vi "Number list to array.vi"(10 "Full names prefix":string, 11 "Number list":string) -> (1 "Comma-separated list":string, 2 "Full names":string[](array[string]), 3 "Number list array":i32[](array[numeric]), 4 "Channlel set":set{i32}(c389))   [LabVIEW 2024, in "File.lvclass"]
uses:
  File/File Class/File.lvclass
  File/File Class/File.lvclass/File.ctl
panel:
  out "repeat channle numbers":bool
  out "substring":string
  out "number":i32
  out "offset past number":i32
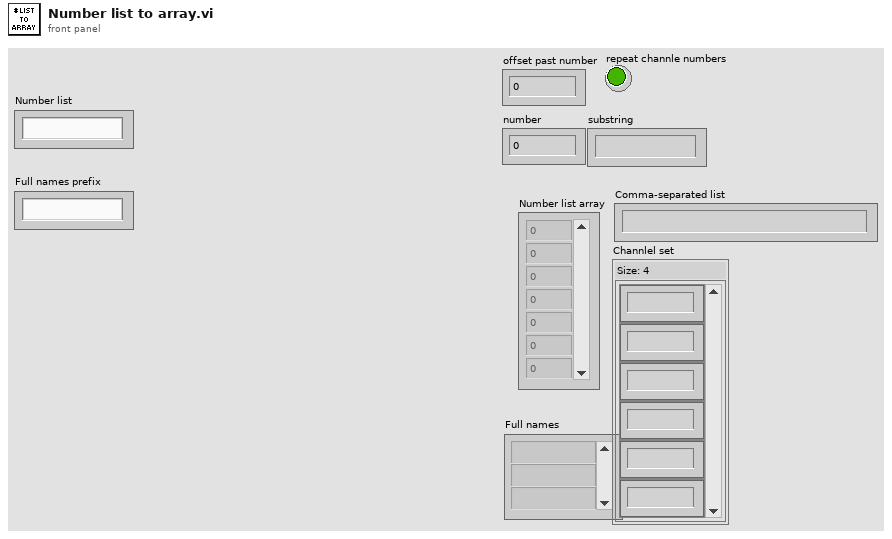
[diagram p1: front panel]
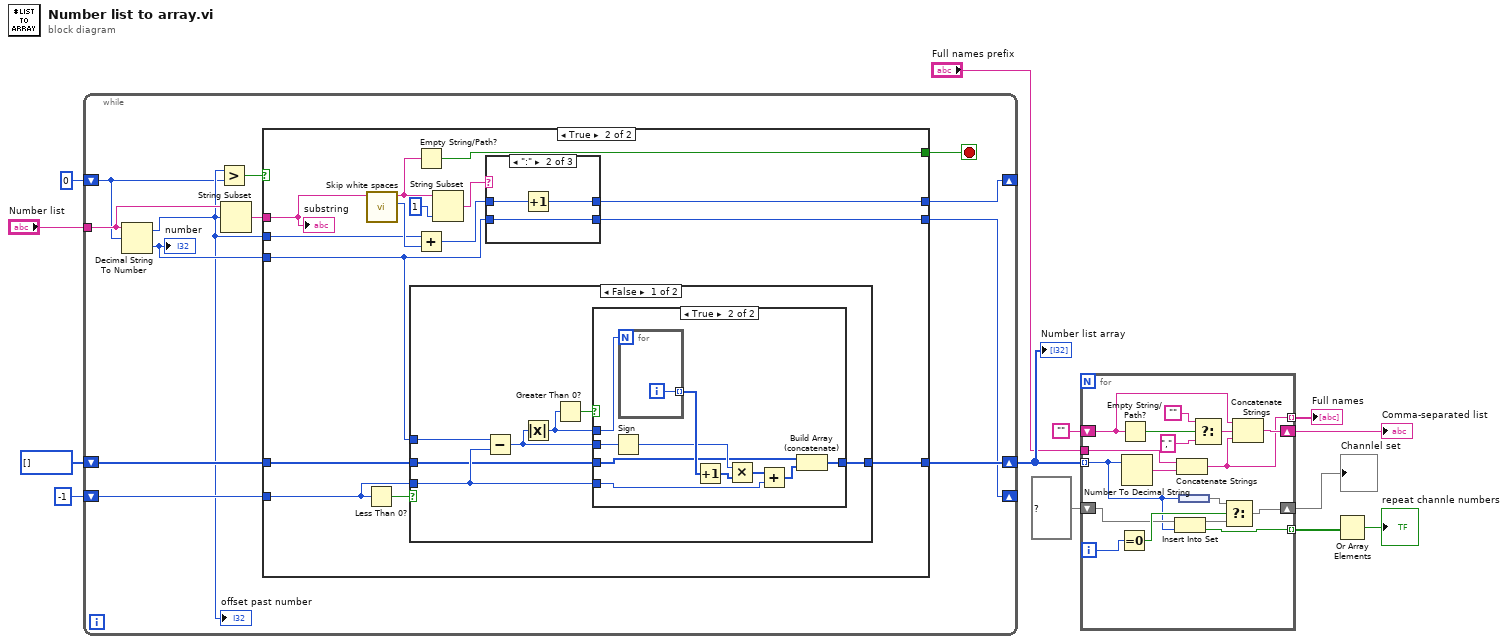
[diagram p0: block diagram]
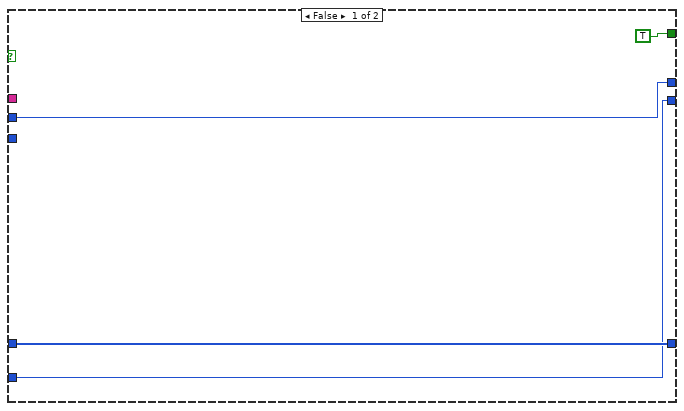
[diagram p2: hidden frame]
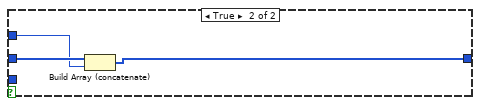
[diagram p4: hidden frame]
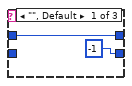
[diagram p5: hidden frame]
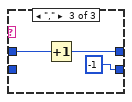
[diagram p6: hidden frame]
diagram:
  n1 = while {
    tunnel: "Number list" -> [w25]
    shift-right: [w17] -> w9
    shift-left: i32[] [] -> [w21]
    shift-right: [w23] -> _
    shift-left: 0 -> [w18]
    shift-right: [w15] -> _
    shift-left: -1 -> [w22]
    stop <- w14 stop-if-true
    n2 = Decimal String To Number(string=w25, offset=w18) -> (offset past number=w19:i32, number=w20:i32)  [unwired: 1 in]
    "offset past number" <- w19
    "number" <- w20
    n3 = Greater?(x=w19, y=w18) -> (0:w16:bool)
    n4 = String Subset(string=w25, offset (0)=w19) -> (substring=w24:string)  [unwired: 1 in]
    n5 = case shown="True" w16 {
      tunnel: w24 -> [_ w44]
      tunnel: [w27 w39] -> w23
      tunnel: w22 -> [w28 w38]
      tunnel: w21 -> [w29 w37]
      tunnel: w20 -> [_ w36]
      tunnel: w19 -> [w27 w35]
      tunnel: [w29 w34] -> w17
      tunnel: [w28 w32] -> w15
      tunnel: [TRUE w31] -> w14
      frame False {
      }
      frame True {
        n6 = Less Than 0?(x=w38) -> (x < 0?=w33:bool)
        n7 = call "Skip white spaces.vi"("String"=w44) -> ("1st non-white space"=w41:i32, "After white spaces"=w30:string)  [unwired: 9 in]
        n8 = case shown="False" w33 {
          tunnel: w37 -> [w48 w66]
          tunnel: [w47 w65] -> w34
          tunnel: w36 -> [w51 w64]
          tunnel: w38 -> [w49 _]
          frame False {
            n9 = Subtract(x=w51, y=w49) -> (x-y=w50:i32)
            n10 = Absolute Value(x=w50) -> (abs(x)=w46:i32)
            n11 = Greater Than 0?(x=w46) -> (x > 0?=w45:bool)
            n12 = case shown="True" w45 {
              tunnel: w50 -> [_ w61]
              tunnel: w46 -> [_ w60]
              tunnel: w49 -> [_ w57]
              tunnel: w48 -> [w52 w54]
              tunnel: [w52 w53] -> w47
              frame False {
              }
              frame True {
                n13 = Sign(1:w61) -> (0:w59:i32)
                n14 = for {
                  N: w60 -> [_]
                  tunnel: [w63] -> w62 mode=indexing
                  i -> [w63]
                }
                n15 = Increment(x=w62) -> (x+1=w58:i32[])
                n16 = Multiply(x=w59, y=w58) -> (x*y=w56:i32[])
                n17 = Add(x=w56, y=w57) -> (x+y=w55:i32[])
                n18 = Build Array (concatenate)(w54, w55) -> (w53:i32[])
              }
            }
          }
          frame True {
            n19 = Build Array (concatenate)(w66, w64) -> (w65:i32[])
          }
        }
        n20 = Empty String/Path?(string/path=w30) -> (empty?=w31:bool)
        n21 = Add(x=w35, y=w41) -> (x+y=w40:i32)
        n22 = String Subset(string=w30, length (rest)=1 ("length (rest)")) -> (substring=w42:string)  [unwired: 1 in]
        n23 = case shown="\":\"" w42 {
          tunnel: w36 -> [_ w69 _]
          tunnel: w40 -> [w68 w71 w74]
          tunnel: [w68 w70 w73] -> w39
          tunnel: [-1 w69 -1] -> w32
          frame "", Default {
          }
          frame ":" {
            n24 = Increment(x=w71) -> (x+1=w70:i32)
          }
          frame "," {
            n25 = Increment(x=w74) -> (x+1=w73:i32)
          }
        }
        "substring" <- w44
      }
    }
  }
  "Number list array" <- w9
  n26 = for {
    tunnel: w9 -> [w76] mode=indexing
    tunnel: [w83] -> w8 mode=indexing
    tunnel: "Full names prefix" -> [w84]
    shift-right: [w86] -> w5
    shift-left: "" -> [w85]
    shift-right: [w79] -> w2
    shift-left: set{i32} {} ("set") -> [w78]
    tunnel: [w75] -> w4 mode=indexing
    i -> [w82]
    n27 = Equal To 0?(x=w82) -> (x = 0?=w80:bool)
    n28 = Empty String/Path?(string/path=w85) -> (empty?=w87:bool)
    n29 = Number To Decimal String(number=w76) -> (decimal integer string=w91:string)  [unwired: 1 in]
    n30 = Insert Into Set(10:w76, 11:w78) -> (2:w75:bool, 3:w77:set{i32})
    n31 = Concatenate Strings(w84, w91) -> (w83:string)
    n32 = node(w76) -> (w81:set{i32})
    n33 = Select(t="", s=w87, f=",") -> (s? t:f=w90:string)
    n34 = Select(t=w81, s=w80, f=w77) -> (s? t:f=w79:set{i32})
    n35 = Concatenate Strings(w85, w90, w83) -> (w86:string)
  }
  "Full names" <- w8
  "Comma-separated list" <- w5
  "Channlel set" <- w2
  n36 = Or Array Elements(Boolean array=w4) -> (logical OR=→"repeat channle numbers":bool)
